vi "SetValue.vi"(8 "error in":errorcluster, 10 "Value":string, 11 "String in":refnum<class "String.lvclass">) -> (0 "error out":errorcluster, 3 "String out":refnum<class "String.lvclass">)   [LabVIEW 2021, in "ProligentXMLGenerator.lvlib" / "String.lvclass"]
uses:
  String.lvclass
  String.lvclass/String.ctl
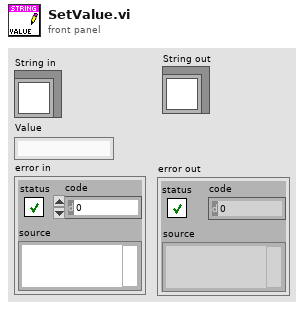
[diagram p1: front panel]
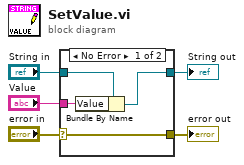
[diagram p0: block diagram]
diagram:
  n1 = case shown="No Error" "error in" {
    selector: "error in" -> [w6 w10]
    tunnel: "String in" -> [w9 w11]
    tunnel: [w8 w11] -> w2
    tunnel: "Value" -> [w7 _]
    tunnel: [w6 w10] -> w1
    frame No Error {
      n2 = Bundle By Name(cluster=w9, "Value"=w7) -> (w8:refnum<class "String.lvclass">)
    }
    frame Error {
    }
  }
  "error out" <- w1
  "String out" <- w2
